vi "send_vehicle_command_float.vi"(2 "brake_amount":sgl, 3 "Drive mode":bool, 4 "error in":errorcluster, 5 "Right amount":dbl, 6 "Forward amount":dbl) -> (0 "error out":errorcluster)   [LabVIEW 2019, in "Lib_Simx.lvlib"]
doc: "Sends a command to the Simulator to control the movement of ego vehicle.\n Parameters:\n -- forward_amount: a value between -1.0 and 1.0 that determines the amount of throttle to apply\n -- right_amount: a value between -1.0 and 1.0 that determines the steering position (-1 is left, +1 is right)\n -- brake_amount: a value between 0.0 and 1.0 that determines the amount of applied brake"
uses:
  Lib_Simx.lvlib
  tools/simx_common.vi
panel:
  out "success":bool
  out "TCP Network Connection out":refnum<k5>
  out "Vehicle command response":string
  # "Overview: Sends a command to the monoDrive Simulator to control the movement of ego vehicle.\n Parameters:\n  -- forward_amount: a value between -1.0 and 1.0 that determines the amount of throttle to apply\n  -- right_amount: a value between -1.0 and 1.0 that determines the steering position (-1 is left, +1 is right)\n  -- brake_amount: a value between 0.0 and 1.0 that determines the amount of applied brake\nInstructions:\nThe command used to control the throttle (forward_amount) and steering (right_amount) is used to move the ego vehicle inside the simulation. The response from the simulator will appear in the vehicle command response field below."
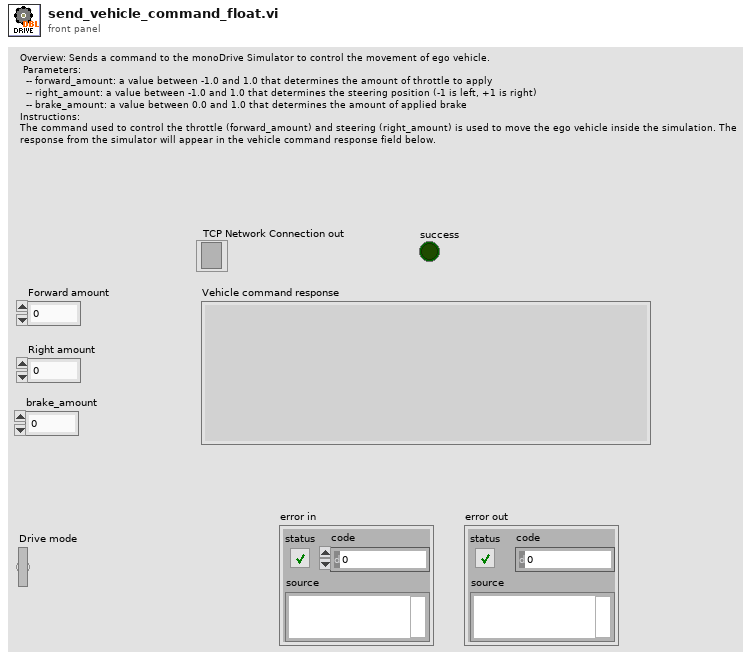
[diagram p1: front panel]
types:
  T1 = typedef "Lib_Simx.lvlib/simx_connection.ctl" = cluster{"Config":T2, "Connections":T5, "Map":cluster{"lanes":cluster{"x":dbl[], "y":dbl[], "z":dbl[]}, "StartPosition":cluster{"start_points":T6, "StartRotation":dbl[], "StartLocation":dbl[]}, "Draw Map Size":T7, "DrawArea":cluster{"min_Y":dbl, "min_X":dbl, "Scale X":dbl, "Scale Y":dbl}, "Map":picture, "Map Geojson":string}}
  T2 = typedef "Lib_Simx.lvlib/config.ctl" = cluster{"Trajectory":T3, "Weather":T4}
  T3 = typedef "Lib_Simx.lvlib/trajectory.ctl" = cluster{"Number of frames":i32, "Frame number":i32, "Trajectory":string}
  T4 = typedef "Lib_Simx.lvlib/weather.ctl" = cluster{"id":string}
  T5 = typedef "Lib_Simx.lvlib/connections.ctl" = cluster{"Simulator Connection":refnum<k5>, "server_ip":string, "Port":i32, "Sensor connections":refnum<k5>[]}
  T6 = typedef "Lib_Simx.lvlib/start_points.ctl" = cluster{"locations":dbl[][], "rotations":dbl[][], "type":string[]}
  T7 = typedef "LVBoundsTypeDef.ctl" = cluster{"Width":u32, "Height":u32}
  T8 = cluster{"forward_amount":dbl, "right_amount":dbl, "brake_amount":sgl, "drive_mode":i16}
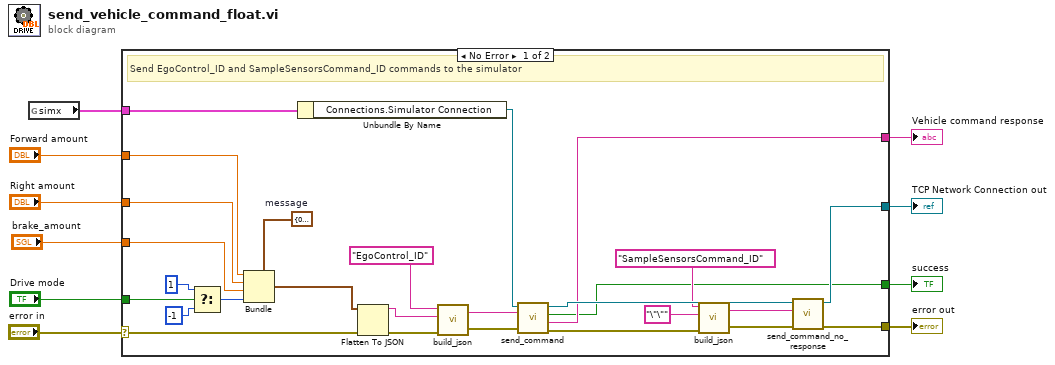
[diagram p0: block diagram]
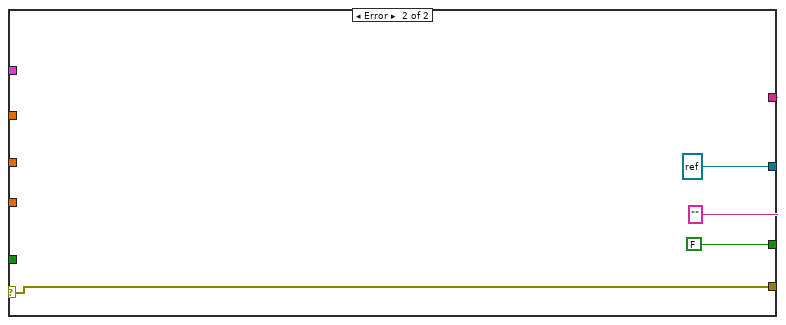
[diagram p2: hidden frame]
diagram:
  n1 = global read "simx_common.vi" "simx"() -> (w2:T1)
  n2 = case shown="No Error" "error in" {
    selector: "error in" -> [w13 w41]
    tunnel: [w25 w41] -> w10
    tunnel: "Right amount" -> [w37 _]
    tunnel: "Forward amount" -> [w36 _]
    tunnel: [w21 "" ("response")] -> w7
    tunnel: [w24 refnum<k5> refnum ("TCP Network Connection Out")] -> w6
    tunnel: [w12 FALSE ("success")] -> w5
    tunnel: "Drive mode" -> [w35 _]
    tunnel: w2 -> [w31 _]
    tunnel: "brake_amount" -> [w11 _]
    frame No Error {
      w14 = T8 {"forward_amount"=0.0, "right_amount"=0.0, "brake_amount"=0.0, "drive_mode"=0}  # message
      # "Send EgoControl_ID and SampleSensorsCommand_ID commands to the simulator"
      n3 = Select(t=1, s=w35, f=-1) -> (s? t:f=w32:i32)
      n4 = Bundle(cluster=w14, "forward_amount"=w36, "right_amount"=w37, "brake_amount"=w11, "drive_mode"=w32) -> (w18:T8)
      n5 = Unbundle By Name(w31) -> ("Connections.Simulator Connection"=w29:refnum<k5>)
      n6 = Flatten To JSON(anything=w18, error in (no error)=w13) -> (JSON string=w16:string, 11:w17:errorcluster)  [unwired: 1 in]
      n7 = call "build_json.vi"("error in"=w17, "Message"=w16, "Command_ID"="EgoControl_ID") -> ("error out"=w30:errorcluster, "JSON Out"=w28:string)  [unwired: 1 in]
      n8 = call "send_command.vi"("error in"=w30, "JSON Command"=w28, "TCP Network Connection in"=w29) -> ("error out"=w27:errorcluster, "Response"=w21:string, "Success"=w12:bool, "TCP Network Connection Out"=w22:refnum<k5>)  [unwired: 1 in]
      n9 = call "build_json.vi"("error in"=w27, "Message"="\"\"" ("message"), "Command_ID"="SampleSensorsCommand_ID" ("type")) -> ("error out"=w26:errorcluster, "JSON Out"=w23:string)  [unwired: 1 in]
      n10 = call "send_command_no_response.vi"("error in"=w26, "JSON Command"=w23, "TCP Network Connection in"=w22) -> ("error out"=w25:errorcluster, "TCP Network Connection Out"=w24:refnum<k5>)  [unwired: 3 in]
    }
    frame Error {
    }
  }
  "Vehicle command response" <- w7
  "TCP Network Connection out" <- w6
  "error out" <- w10
  "success" <- w5
